vi "Create Cron Job.vi"(5 "Cron in":refnum<class "Cron.lvclass">, 8 "error in (no error)":errorcluster, 11 "Cron Expression":string) -> (0 "error out":errorcluster, 1 "expression valid":bool, 3 "Cron out":refnum<class "Cron.lvclass">)   [LabVIEW 2013, in "openCron.lvlib" / "Cron.lvclass"]
uses:
  Cron.lvclass
  Cron.lvclass/Cron.ctl
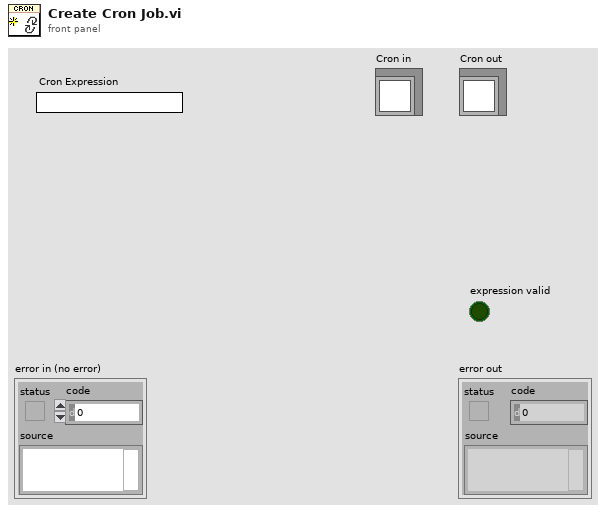
[diagram p1: front panel]
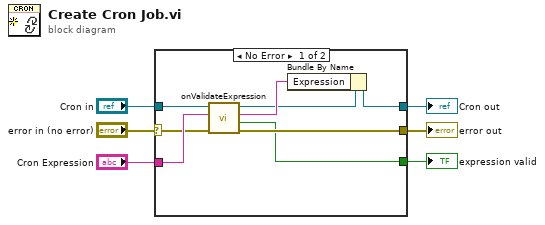
[diagram p0: block diagram]
diagram:
  n1 = case shown="No Error" "error in (no error)" {
    selector: "error in (no error)" -> [w12 w16]
    tunnel: [w11 w16] -> w5
    tunnel: [w7 w15] -> w3
    tunnel: "Cron in" -> [w14 w15]
    tunnel: "Cron Expression" -> [w13 _]
    tunnel: [w10 _] -> w1
    frame No Error {
      n2 = call-dynamic "onValidateExpression.vi"("error in (no error)"=w12, "Expression"=w13, "Cron in"=w14) -> ("error out"=w11:errorcluster, "valid?"=w10:bool, "Validated Expression"=w9:string, "Cron out"=w8:refnum<class "Cron.lvclass">)  [unwired: 5 in]
      n3 = Bundle By Name(cluster=w8, "Expression"=w9) -> (w7:refnum<class "Cron.lvclass">)
    }
    frame Error {
    }
  }
  "error out" <- w5
  "Cron out" <- w3
  "expression valid" <- w1
